vi "Handle getAll.vi"(8 "error in (no error)":errorcluster, 11 "Inst.Magneto in":refnum<class "Inst.Magneto.lvclass">) -> (0 "error out":errorcluster, 2 "getAll":variant, 3 "Inst.Magneto out":refnum<class "Inst.Magneto.lvclass">)   [LabVIEW 2019, in "Inst.Magneto.lvclass"]
uses:
  Inst.Magneto.lvclass
  Inst.Magneto.lvclass/Inst.Magneto.ctl
  Typedefs/Inst.Magneto.getAll--Cluster.ctl
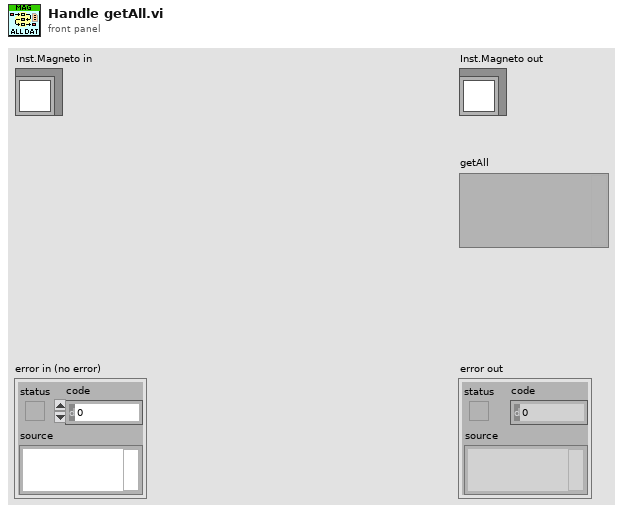
[diagram p1: front panel]
types:
  T1 = typedef "Inst.Magneto.lvclass/Inst.Magneto.getAll--Cluster.ctl" = cluster{"AllString":string}
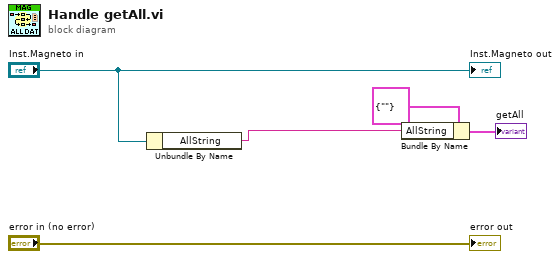
[diagram p0: block diagram]
diagram:
  n1 = Unbundle By Name("Inst.Magneto in") -> ("AllString"=w1:string)
  n2 = Bundle By Name(cluster=T1 {"AllString"=""} ("getAll"), "AllString"=w1) -> (→"getAll":T1)
  "error out" <- "error in (no error)"
  "Inst.Magneto out" <- "Inst.Magneto in"
